vi "BK Precision 1823A Monitor Frequency.vi"() -> ()   [LabVIEW 2017]
doc: "This exampleis used to monitor the measurement values obtained from B&K Precision 1823A frequency counter."
uses:
  BK Precision 1823A.lvlib
panel:
  in  "Update Time (1000)":u16=1000 min=100 step=1
  out "Measured Data Value":string
  in  "Select Function":i8(ring) items=["Frequency A", "Frequency B", "Frequency C", "Period", "Total", "Ratio", "T.I"]
  in  "Select Gate Time":i8(ring) items=["0.01", "0.1", "1", "10"]
  in  "stop":bool
  in  "VISA resource name":refnum<visa-resource-name>
  # "(c) 2009 B&K PRECISION CORPORATION.  ALL RIGHTS RESERVED."
  # "ms"
  # "seconds"
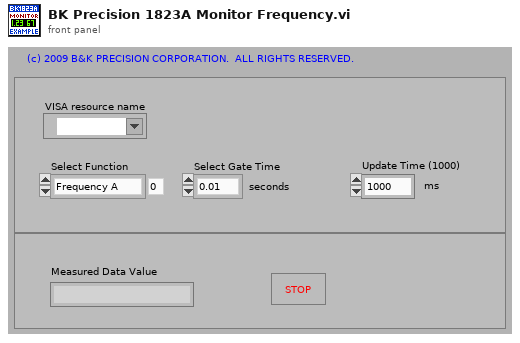
[diagram p1: front panel]
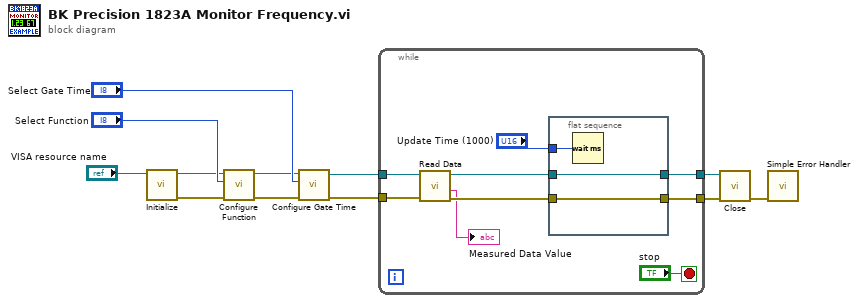
[diagram p0: block diagram]
diagram:
  n1 = call "Initialize.vi"("VISA resource name"="VISA resource name") -> ("error out"=w3:errorcluster, "VISA resource name out"=w4:refnum<visa-resource-name>)  [unwired: 9 in]
  n2 = call "Configure Function.vi"("error in (no error)"=w3, "Select Function (0)"="Select Function", "VISA resource name"=w4) -> ("error out"=w1:errorcluster, "VISA resource name out"=w2:refnum<visa-resource-name>)  [unwired: 7 in]
  n3 = call "Configure Gate Time.vi"("error in (no error)"=w1, "Select Gate Time (0.01)"="Select Gate Time", "VISA resource name"=w2) -> ("error out"=w8:errorcluster, "VISA resource name out"=w9:refnum<visa-resource-name>)  [unwired: 7 in]
  n4 = while {
    tunnel: [w19] -> w11
    tunnel: [w17] -> w10
    tunnel: w9 -> [w15]
    tunnel: w8 -> [w14]
    stop <- "stop" stop-if-true
    n5 = call "Read Data.vi"("error in (no error)"=w14, "VISA resource name"=w15) -> ("error out"=w16:errorcluster, "Return String"=→"Measured Data Value":string, "VISA resource name out"=w18:refnum<visa-resource-name>)  [unwired: 6 in, 1 out]
    n6 = flat-sequence {
      tunnel: "Update Time (1000)" -> [w24]
      tunnel: [w23] -> w19
      tunnel: w18 -> [w23]
      tunnel: [w22] -> w17
      tunnel: w16 -> [w22]
      frame #0 {
        n7 = Wait (ms)(milliseconds to wait=w24) -> ()  [unwired: 1 out]
      }
    }
  }
  n8 = call "Close.vi"("error in (no error)"=w10, "VISA resource name"=w11) -> ("error out"=w12:errorcluster)  [unwired: 9 in]
  n9 = call <vilib>:"Simple Error Handler.vi"("error in (no error)"=w12) -> ()  [unwired: 4 in, 5 out]
